vi "I3252_Edit_Setpoint.vi"(1 "Read String":string) -> (0 "Setpoint is":dbl)   [LabVIEW 2013]
panel:
  in  "Comma":T1(ring)
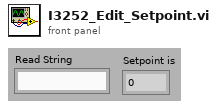
[diagram p1: front panel]
types:
  T1 = enum16{"0", "1", "2", "3", "4", "8", "9", "A", "B", "C"}
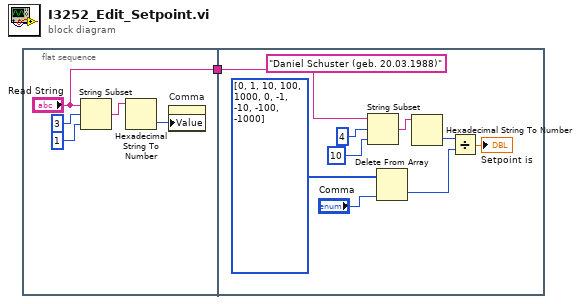
[diagram p0: block diagram]
diagram:
  (unwired) "Daniel Schuster (geb. 20.03.1988)"
  n1 = flat-sequence {
    tunnel: ["Read String"] -> w1
    tunnel: w1 -> [w8]
    frame #0 {
      n2 = String Subset(string="Read String", offset (0)=3, length (rest)=1 ("length (rest)")) -> (substring=w5:string)
      n3 = Hexadecimal String To Number(string=w5) -> (number=w6:u32)  [unwired: 2 in, 1 out]
      n4 = property on="Comma" class="Enum (strict)"("Value"=w6) -> ()  [unwired: 2 in, 2 out]
    }
    frame #1 {
      n5 = String Subset(string=w8, offset (0)=4, length (rest)=10) -> (substring=w13:string)
      n6 = Delete From Array(array=i32[] [0, 1, 10, 100, 1000, 0, -1, -10, -100, -1000] ("Array"), index="Comma") -> (deleted portion=w9:i32)  [unwired: 1 in, 1 out]
      n7 = Hexadecimal String To Number(string=w13) -> (number=w12:u32)  [unwired: 2 in, 1 out]
      n8 = Divide(x=w12, y=w9) -> (x/y=→"Setpoint is":dbl)
    }
  }
